vi "Digital Event Constructor.vi"(8 "error in (no error)":errorcluster, 10 "Capture Path":path, 11 "Signal Parameters":string) -> (0 "error out":errorcluster, 3 "Digital Event.lvclass":refnum<class "Digital Event.lvclass">)   [LabVIEW 2015, in "Digital Event.lvclass"]
uses:
  Digital Event.lvclass
  Digital Event.lvclass/Digital Event.ctl
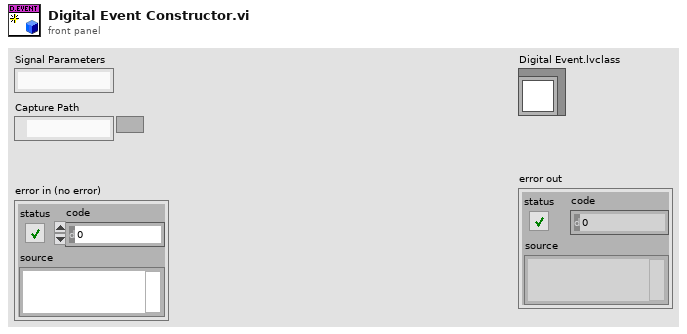
[diagram p1: front panel]
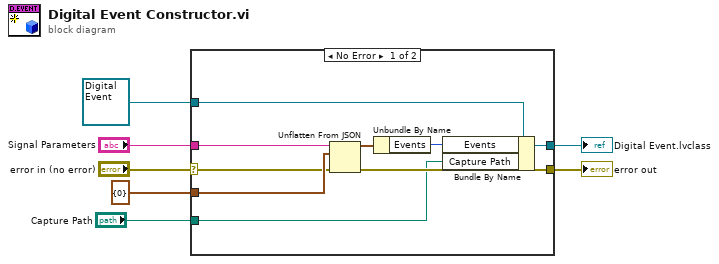
[diagram p0: block diagram]
diagram:
  n1 = case shown="No Error" "error in (no error)" {
    selector: "error in (no error)" -> [w9 w18]
    tunnel: refnum<class "Digital Event.lvclass"> refnum ("Digital Event.lvclass") -> [w16 w17]
    tunnel: [w15 w17] -> w6
    tunnel: "Signal Parameters" -> [w14 _]
    tunnel: cluster{"Events":u32} {"Events"=0} -> [w13 _]
    tunnel: [w12 w18] -> w3
    tunnel: "Capture Path" -> [w8 _]
    frame No Error {
      n2 = Unflatten From JSON(JSON string=w14, type and defaults=w13, error in (no error)=w9) -> (value=w11:cluster{"Events":u32}, error out=w12:errorcluster)  [unwired: 4 in]
      n3 = Unbundle By Name(w11) -> ("Events"=w10:u32)
      n4 = Bundle By Name(cluster=w16, "Events"=w10, "Capture Path"=w8) -> (w15:refnum<class "Digital Event.lvclass">)
    }
    frame Error {
    }
  }
  "Digital Event.lvclass" <- w6
  "error out" <- w3
